vi "Open Audio FGV.vi"(6 "Command":T1, 8 "Open?":bool) -> (0 "Open":bool)   [LabVIEW 2015]
uses:
  TypeDefs Host/Open Audio FGV Enum.ctl
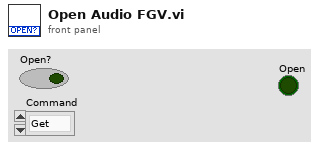
[diagram p1: front panel]
types:
  T1 = typedef "Open Audio FGV Enum.ctl" = enum16{"Get", "Set"}
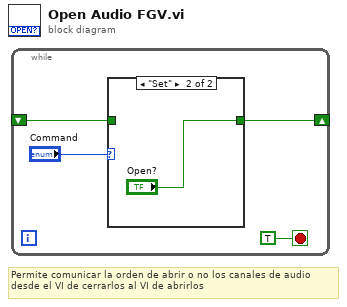
[diagram p0: block diagram]
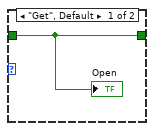
[diagram p2: hidden frame]
diagram:
  # "Permite comunicar la orden de abrir o no los canales de audio\ndesde el VI de cerrarlos al VI de abrirlos"
  n1 = while {
    shift-right: [w2] -> _
    shift-left: _ -> [w1]
    stop <- TRUE stop-if-true
    n2 = case shown="\"Set\"" "Command" {
      tunnel: [w5 "Open?"] -> w2
      tunnel: w1 -> [w5 _]
      frame "Get", Default {
        "Open" <- w5
      }
      frame "Set" {
      }
    }
  }
